vi "ServoControl.vi"(10 "Servo data in":T2, 11 "UI Data":T1) -> ()   [LabVIEW 2023]
uses:
  controls/ServoData.ctl
  controls/UI Data.ctl
  maestro/Maestro.lvlib
panel:
  out "Name":string
  in  "Target":u16(slide) scale=400.0..2000.0
  out "Channel":u8
  in  "Stop Button":bool
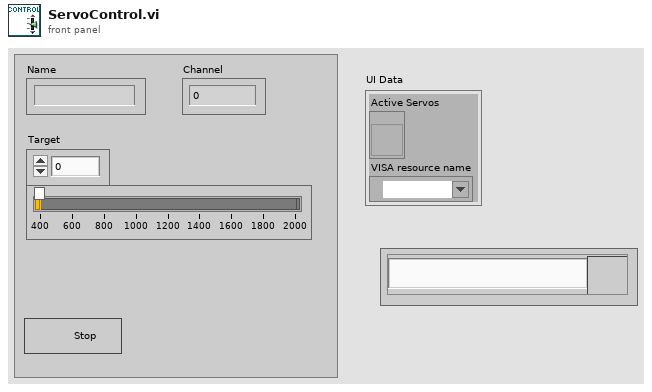
[diagram p1: front panel]
types:
  T1 = typedef "UI Data.ctl" = cluster{"Active Servos":refnum<vi>, "VISA resource name":refnum<visa-resource-name>}
  T2 = typedef "ServoData.ctl" = cluster{"Name":string, "Channel":u8, "Delete Button":bool}
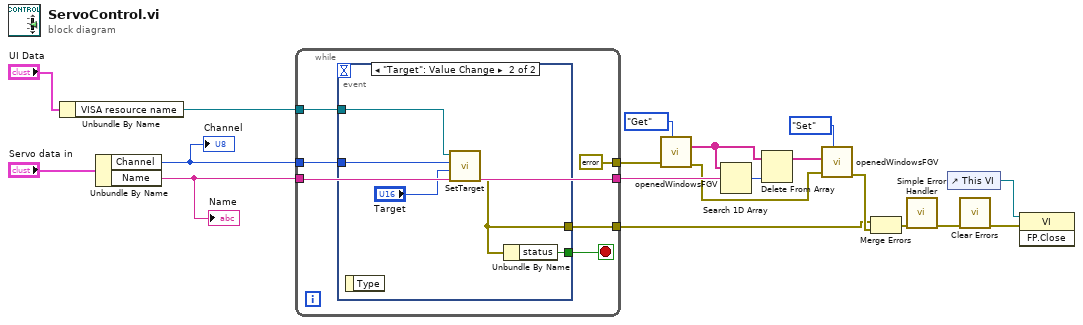
[diagram p0: block diagram]
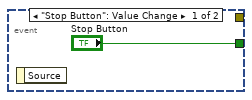
[diagram p2: hidden frame]
diagram:
  n1 = Unbundle By Name("UI Data") -> ("VISA resource name"=w17:refnum<visa-resource-name>)
  n2 = Unbundle By Name("Servo data in") -> ("Channel"=w13:u8, "Name"=w12:string)
  "Channel" <- w13
  "Name" <- w12
  n3 = while {
    tunnel: [w24] -> w2
    tunnel: w13 -> [w22]
    tunnel: w17 -> [w23]
    tunnel: w12 -> [w21]
    tunnel: [w21] -> w8
    tunnel: [errorcluster {"status"=FALSE, "code"=0, "source"=""} ("error in")] -> w1
    stop <- w25 stop-if-true
    n4 = event shown="[1] \"Target\": Value Change" {
      selector: _ -> [_ _]
      dyn-events: _ -> [_ _]
      timeout: _ -> [_ _]
      tunnel: ["Stop Button" w27] -> w25
      tunnel: [_ w28] -> w24
      tunnel: w23 -> [_ w31]
      tunnel: w22 -> [_ w30]
      event "Stop Button": Value Change {
        n5 = event-data() -> ()  [unwired: 1 in, 1 out]
      }
      event "Target": Value Change {
        n6 = event-data() -> ()  [unwired: 1 in, 1 out]
        n7 = call "SetTarget.vi"("Position"="Target", "Channel"=w30, "VISA resource name"=w31) -> ("error out"=w28:errorcluster)  [unwired: 7 in, 1 out]
        n8 = Unbundle By Name(w28) -> ("status"=w27:bool)
      }
    }
  }
  n9 = call "openedWindowsFGV.vi"("Action"=enum16{"Get", "Set"}."Get", "error in"=w1) -> ("error out"=w5:errorcluster, "Names out"=w10:string[])  [unwired: 8 in]
  n10 = Search 1D Array(1D array=w10, element=w8) -> (index of element=w9:i32)  [unwired: 1 in]
  n11 = Delete From Array(array=w10, index=w9) -> (array with subset deleted=w11:string[])  [unwired: 1 in, 1 out]
  n12 = call "openedWindowsFGV.vi"("Action"=enum16{"Get", "Set"}."Set", "error in"=w5, "Names in"=w11) -> ("error out"=w3:errorcluster)  [unwired: 7 in, 1 out]
  n13 = Merge Errors(w2, w3) -> (w4:errorcluster)
  n14 = call <vilib>:"Simple Error Handler.vi"("error in (no error)"=w4) -> ("error out"=w16:errorcluster)  [unwired: 4 in, 4 out]
  n15 = control-ref of="This VI"() -> (w14:refnum<vi>)
  n16 = call <vilib>:"Clear Errors.vi"("error in (no error)"=w16) -> ("error out"=w15:errorcluster)  [unwired: 5 in, 1 out]
  n17 = invoke class="VI" method="FP.Close"(reference=w14, error in=w15) -> ()  [unwired: 1 in, 3 out]
